vi "反馈拼接.vi"(0 "反馈参数":T1) -> (14 "计算后字符串":string)   [LabVIEW 2019, in "MainPage.lvlib" / "MainPage.lvclass"]
uses:
  MainPage.lvclass
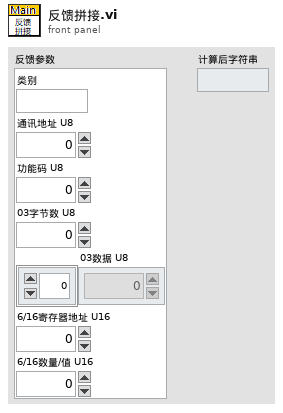
[diagram p1: front panel]
types:
  T1 = cluster{"类别":string, "通讯地址 U8":u8, "功能码 U8":u8, "03字节数 U8":u8, "03数据 U8":u8[], "6/16寄存器地址 U16":u16, "6/16数量/值 U16":u16}
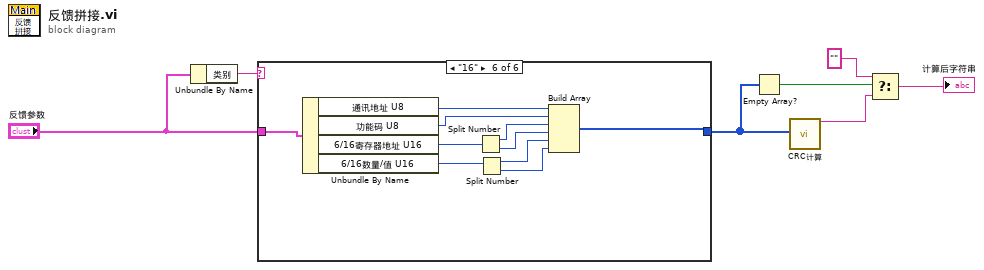
[diagram p0: block diagram]
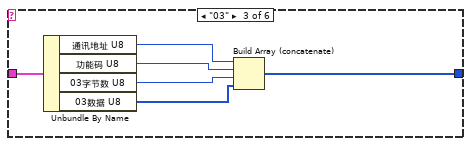
[diagram p4: hidden frame]
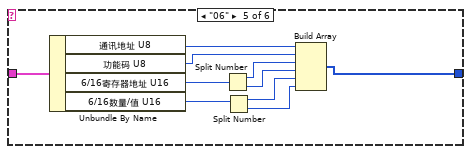
[diagram p6: hidden frame]
diagram:
  n1 = Unbundle By Name("反馈参数") -> ("类别"=w1:string)
  n2 = case shown="\"16\"" w1 {
    tunnel: "反馈参数" -> [_ _ w13 _ w23 w25]
    tunnel: [_ _ w8 _ w14 w24] -> w3
    frame Default {
    }
    frame "未知" {
    }
    frame "03" {
      n3 = Unbundle By Name(w13) -> ("通讯地址 U8"=w12:u8, "功能码 U8"=w11:u8, "03字节数 U8"=w10:u8, "03数据 U8"=w9:u8[])
      n4 = Build Array (concatenate)(w12, w11, w10, w9) -> (w8:u8[])
    }
    frame "05" {
    }
    frame "06" {
      n5 = Unbundle By Name(w23) -> ("通讯地址 U8"=w20:u8, "功能码 U8"=w19:u8, "6/16寄存器地址 U16"=w22:u16, "6/16数量/值 U16"=w21:u16)
      n6 = Split Number(x=w22) -> (hi(x)=w18:u8, lo(x)=w17:u8)
      n7 = Split Number(x=w21) -> (hi(x)=w16:u8, lo(x)=w15:u8)
      n8 = Build Array(w20, w19, w18, w17, w16, w15) -> (w14:u8[])
    }
    frame "16" {
      n9 = Unbundle By Name(w25) -> ("通讯地址 U8"=w31:u8, "功能码 U8"=w30:u8, "6/16寄存器地址 U16"=w33:u16, "6/16数量/值 U16"=w32:u16)
      n10 = Split Number(x=w33) -> (hi(x)=w29:u8, lo(x)=w28:u8)
      n11 = Split Number(x=w32) -> (hi(x)=w27:u8, lo(x)=w26:u8)
      n12 = Build Array(w31, w30, w29, w28, w27, w26) -> (w24:u8[])
    }
  }
  n13 = Empty Array?(array=w3) -> (empty?=w4:bool)
  n14 = call "CRC计算.vi"("无校验U8数组"=w3) -> ("计算后字符串"=w5:string)  [unwired: 17 in, 1 out]
  n15 = Select(t="", s=w4, f=w5) -> (s? t:f=→"计算后字符串":string)
